vi "Wind Speed to Rotation Speed Simulation.vi"(11 "Wind Speed":dbl) -> (3 "Numeric":dbl)   [LabVIEW 2009]
doc: "This simplified VI inputs the wind speed and outputs what could be the rotation associated with wind speed. It is not a true simulation. For a real world simulation that incorporates many aspects of a Wind Turbine see www.ni.com.\n\nAAL 9/09"
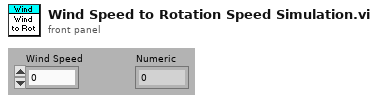
[diagram p1: front panel]
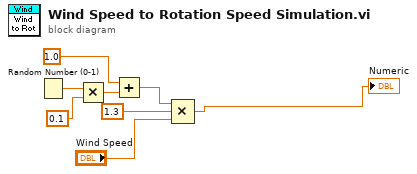
[diagram p0: block diagram]
diagram:
  n1 = Random Number (0-1)() -> (number: 0 to 1=w1:dbl)
  n2 = Multiply(x=w1, y=0.1) -> (x*y=w4:dbl)
  n3 = Add(x=1.0, y=w4) -> (x+y=w7:dbl)
  n4 = Compound Arithmetic op=MULTIPLY(w7, 1.3 ("y"), "Wind Speed") -> (→"Numeric":dbl)
